vi "Demo.vi"(8 "error in (no error)":errorcluster) -> (0 "error out":errorcluster, 3 "directory copy":path)   [LabVIEW 2019]
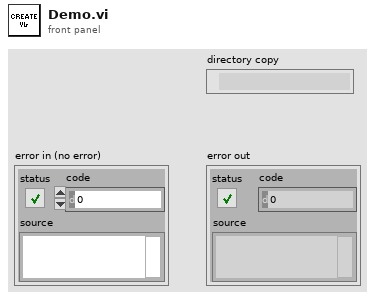
[diagram p1: front panel]
types:
  T1 = cluster{"left":i16, "top":i16, "right":i16, "bottom":i16}
  T2 = typedef "imagedata.ctl" = cluster{"image type":i32, "image depth":i32, "image":u8[], "mask":u8[], "colors":u32[], "Rectangle":cluster{"left":i16, "top":i16, "right":i16, "bottom":i16}}
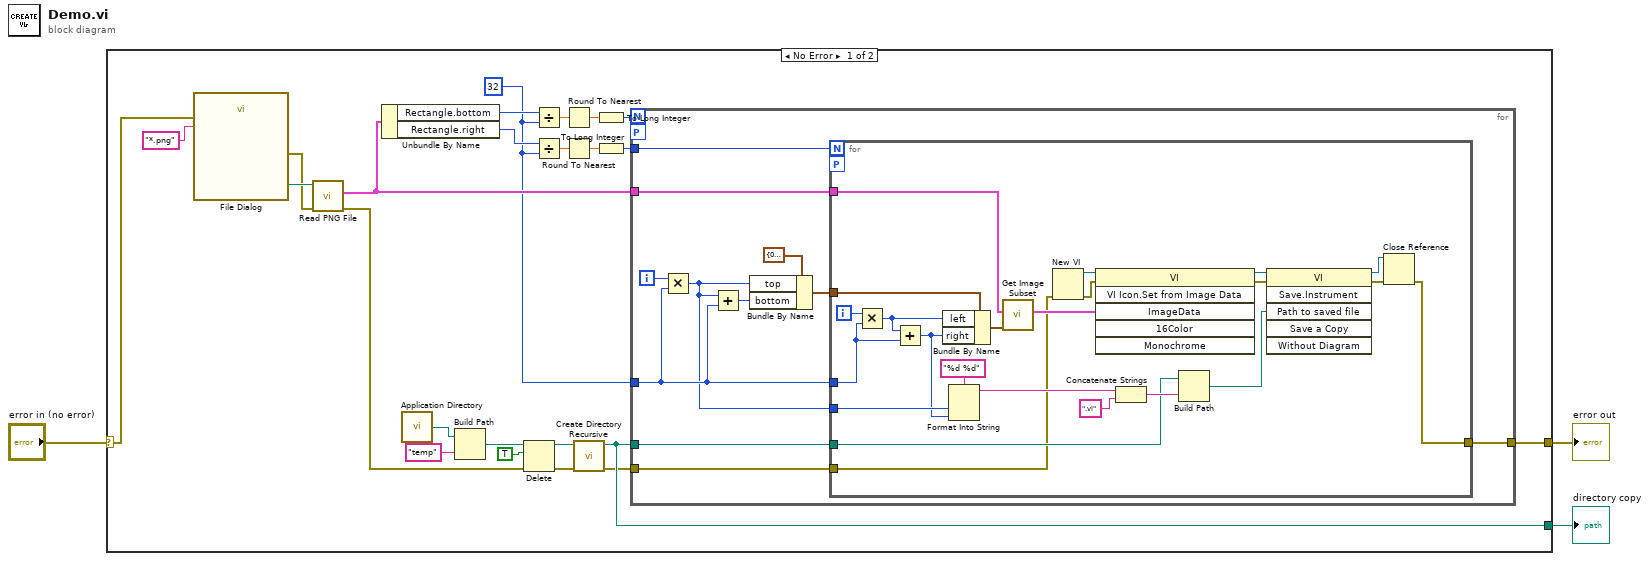
[diagram p0: block diagram]
diagram:
  n1 = case shown="No Error" "error in (no error)" {
    selector: "error in (no error)" -> [w5 w62]
    tunnel: [w15 _] -> w3
    tunnel: [w4 w62] -> w1
    frame No Error {
      w13 = i16 32 ("y")
      n2 = call "File Dialog"("error in"=w5, "pattern (all files)"="*.png") -> ("selected path"=w22:path, "error out"=w9:errorcluster)  [unwired: 10 in, 2 out]
      n3 = call <vilib>:"Read PNG File.vi"("error in (no error)"=w9, "path to PNG file"=w22) -> ("error out"=w8:errorcluster, "image data"=w27:T2)  [unwired: 7 in, 1 out]
      n4 = Unbundle By Name(w27) -> ("Rectangle.bottom"=w26:i16, "Rectangle.right"=w14:i16)
      n5 = call <vilib>:"Application Directory.vi"() -> ("Application Directory"=w18:path)
      n6 = Build Path(base path=w18, name or relative path="temp") -> (appended path=w19:path)
      n7 = Delete(path (use dialog)=w19, entire hierarchy (F)=TRUE, error in=w8) -> (deleted path=w20:path, error out=w7:errorcluster)  [unwired: 2 in, 1 out]
      n8 = Divide(x=w26, y=w13) -> (x/y=w24:dbl)
      n9 = Divide(x=w14, y=w13) -> (x/y=w25:dbl)
      n10 = Round To Nearest(number=w24) -> (nearest integer value=w12:dbl)
      n11 = Round To Nearest(number=w25) -> (nearest integer value=w23:dbl)
      n12 = call <vilib>:"Create Directory Recursive.vi"("error in (no error)"=w7, "directory"=w20) -> ("error out"=w6:errorcluster, "directory copy"=w15:path)  [unwired: 3 in, 1 out]
      n13 = To Long Integer(number=w12) -> (32bit integer=w11:i32)
      n14 = To Long Integer(number=w23) -> (32bit integer=w10:i32)
      n15 = for {
        N: w11 -> [_]
        tunnel: w27 -> [w38]
        tunnel: w10 -> [w37]
        tunnel: w13 -> [w34]
        tunnel: w15 -> [w31]
        workers-P: _ -> [_]
        tunnel: w6 -> [w29]
        tunnel: [w28] -> w4
        i -> [w35]
        n16 = Multiply(x=w35, y=w34) -> (x*y=w32:i32)
        n17 = Add(x=w32, y=w34) -> (x+y=w33:i32)
        n18 = Bundle By Name(cluster=T1 {"left"=0, "top"=0, "right"=0, "bottom"=0} ("subset rect"), "top"=w32, "bottom"=w33) -> (w36:T1)
        n19 = for {
          N: w37 -> [_]
          tunnel: w36 -> [w61]
          tunnel: w38 -> [w60]
          tunnel: w34 -> [w58]
          tunnel: w32 -> [w45]
          tunnel: w31 -> [w42]
          workers-P: _ -> [_]
          tunnel: w29 -> [w41]
          tunnel: [w39] -> w28
          i -> [w59]
          n20 = Multiply(x=w59, y=w58) -> (x*y=w44:i32)
          n21 = Add(x=w44, y=w58) -> (x+y=w43:i32)
          n22 = Bundle By Name(cluster=w61, "left"=w44, "right"=w43) -> (w48:T1)
          n23 = Format Into String(format string="%d %d", w45, w43) -> (resulting string=w46:string)  [unwired: 2 in, 1 out]
          n24 = call <vilib>:"Get Image Subset.vi"("subset rect"=w48, "image data"=w60) -> ("image subset"=w56:T2)  [unwired: 4 in, 1 out]
          n25 = New VI(8:w41) -> (0:w40:errorcluster, 3:w57:refnum<vi>)  [unwired: 6 in]
          n26 = invoke class="VI" method="VI Icon.Set from Image Data"(reference=w57, error in=w40, "ImageData"=w56) -> (reference out=w55:refnum<vi>, error out=w51:errorcluster)  [unwired: 3 in, 4 out]
          n27 = Concatenate Strings(w46, ".vi" ("string")) -> (w54:string)
          n28 = Build Path(base path=w42, name or relative path=w54) -> (appended path=w52:path)
          n29 = invoke class="VI" method="Save.Instrument"(reference=w55, error in=w51, "Path to saved file"=w52) -> (reference out=w50:refnum<vi>, error out=w49:errorcluster)  [unwired: 3 in, 4 out]
          n30 = Close Reference(reference=w50, error in (no error)=w49) -> (error out=w39:errorcluster)
        }
      }
    }
    frame Error {
    }
  }
  "error out" <- w1
  "directory copy" <- w3
